vi "Agilent MXA Series List Sweep.vi"() -> ()   [LabVIEW 2018]
doc: "This example shows how to configure the spectrum analyzer under List Sweep mode and acquire the measurement data."
uses:
  Agilent MXA Series.lvlib
panel:
  in  "Timeout (10000 ms)":i32=10000 format="%.0g"
  out "Measurement Data":dbl[](array[numeric])
  in  "Detector List":i32[](array[ring])=[0, 0, 0] items=["LAVG", "VAVG", "RMS", "Negative", "Positive", "Sample", "Peak-AVER", "Peak-RMS", "DualAvg"]
  in  "Mechanical Attenuator List":dbl[](array[numeric])=[10.0, 10.0, 10.0]
  in  "Frequency List":dbl[](array[numeric])=[1000000000.0, 1000000000.0, 1000000000.0]
  in  "VISA resource name":refnum<visa-resource-name>
  # "(c) 2007-2015 National Instruments.  ALL RIGHTS RESERVED."
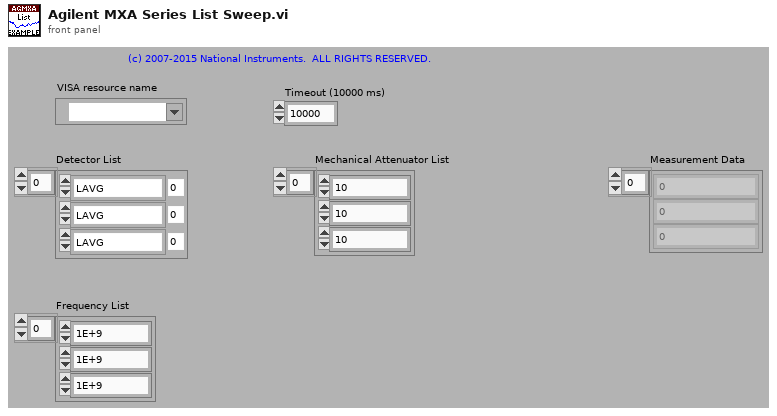
[diagram p1: front panel]
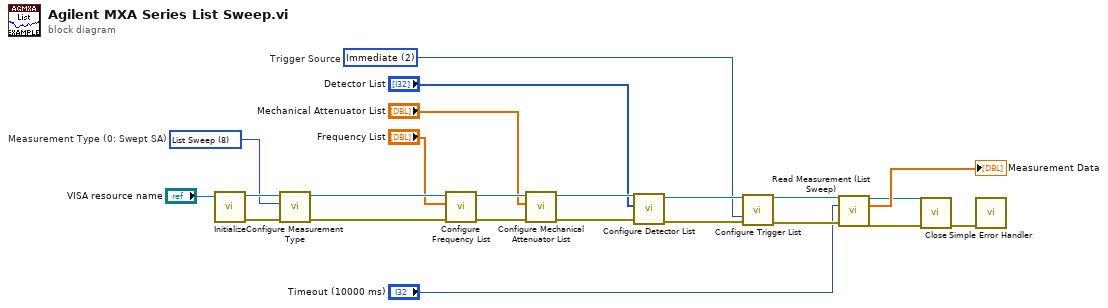
[diagram p0: block diagram]
diagram:
  w7 = 2 items=["External1", "External2", "Immediate", "BUS"]  # Trigger Source
  w19 = 8 items=["Swept SA", "Channel Power", "Occupied Bandwidth", "Power Stat CCDF", "Adjacent Channel Power", "Burst Power", "Spurious Emissions", "Spectrum Emission Mask", "List Sweep"]  # Measurement Type (0: Swept SA)
  n1 = call "Initialize.vi"("VISA resource name"="VISA resource name") -> ("error out"=w20:errorcluster, "VISA resource name out"=w21:refnum<visa-resource-name>)  [unwired: 9 in]
  n2 = call "Configure Measurement Type.vi"("error in (no error)"=w20, "Measurement Type (0: Swept SA)"=w19, "VISA resource name"=w21) -> ("error out"=w17:errorcluster, "VISA resource name out"=w18:refnum<visa-resource-name>)  [unwired: 7 in]
  n3 = call "Configure Frequency List.vi"("error in (no error)"=w17, "Frequency List"="Frequency List", "VISA resource name"=w18) -> ("error out"=w14:errorcluster, "VISA resource name out"=w15:refnum<visa-resource-name>)  [unwired: 7 in]
  n4 = call "Configure Mechanical Attenuator List.vi"("error in (no error)"=w14, "Mechanical Attenuator List"="Mechanical Attenuator List", "VISA resource name"=w15) -> ("error out"=w11:errorcluster, "VISA resource name out"=w12:refnum<visa-resource-name>)  [unwired: 7 in]
  n5 = call "Configure Detector List.vi"("error in (no error)"=w11, "Detector List"="Detector List", "VISA resource name"=w12) -> ("error out"=w8:errorcluster, "VISA resource name out"=w9:refnum<visa-resource-name>)  [unwired: 7 in]
  n6 = call "Configure Trigger List.vi"("VISA resource name"=w9, "Trigger Source"=w7, "error in (no error)"=w8) -> ("VISA resource name out"=w6:refnum<visa-resource-name>, "error out"=w5:errorcluster)  [unwired: 11 in]
  n7 = call "Read Measurement (List Sweep).vi"("VISA resource name"=w6, "Timeout (10000 ms)"="Timeout (10000 ms)", "error in (no error)"=w5) -> ("VISA resource name out"=w2:refnum<visa-resource-name>, "Measurement Data"=→"Measurement Data":dbl[], "error out"=w3:errorcluster)  [unwired: 10 in]
  n8 = call "Close.vi"("error in (no error)"=w3, "VISA resource name"=w2) -> ("error out"=w23:errorcluster)  [unwired: 9 in]
  n9 = call <vilib>:"Simple Error Handler.vi"("error in (no error)"=w23) -> ()  [unwired: 4 in, 5 out]
